vi "SimpleProducerConsumer.vi"() -> ()   [LabVIEW 2014]
doc: "This example shows a simple Producer Consumer implementation on the RasPi\ntarget. Enter Command to be sent on the String control. By pressing the\nSend button, command is sent from Producer loop and shows up on the Message Received indicator that is updated on the Consumer loop. The Count indicator updates the number of iterations the Consumer loop executes.\nSend stop command to stop both parallel loops and quit the VI."
panel:
  out "Count":i32
  out "Message Received":string
  in  "Send":bool
  in  "String":string
  # "Pass 'stop' to end program"
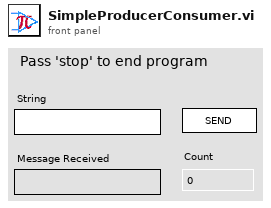
[diagram p1: front panel]
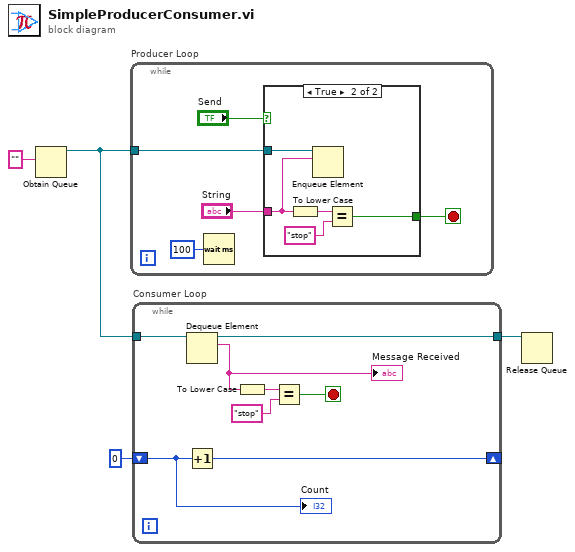
[diagram p0: block diagram]
diagram:
  n1 = Obtain Queue(element data type="") -> (queue out=w2:refnum<queue>)  [unwired: 4 in, 2 out]
  n2 = while "Producer Loop" {
    tunnel: w2 -> [w7]
    stop <- w5 stop-if-true
    n3 = Wait (ms)(milliseconds to wait=u32 100) -> ()  [unwired: 1 out]
    n4 = case shown="True" "Send" {
      tunnel: w7 -> [_ w14]
      tunnel: "String" -> [_ w13]
      tunnel: [_ w10] -> w5
      frame False {
      }
      frame True {
        n5 = To Lower Case(string=w13) -> (all lower case string=w11:string)
        n6 = Enqueue Element(queue=w14, element=w13) -> ()  [unwired: 2 in, 3 out]
        n7 = Equal?(x=w11, y="stop") -> (x = y?=w10:bool)
      }
    }
  }
  n8 = while "Consumer Loop" {
    shift-right: [w21] -> _
    shift-left: 0 -> [w15]
    tunnel: w2 -> [w22]
    tunnel: [w16] -> w1
    stop <- w17 stop-if-true
    n9 = Dequeue Element(queue=w22) -> (queue out=w16:refnum<queue>, element=w18:string)  [unwired: 2 in, 2 out]
    "Message Received" <- w18
    n10 = Increment(x=w15) -> (x+1=w21:i32)
    n11 = To Lower Case(string=w18) -> (all lower case string=w20:string)
    n12 = Equal?(x=w20, y="stop") -> (x = y?=w17:bool)
    "Count" <- w15
  }
  n13 = Release Queue(queue=w1) -> ()  [unwired: 2 in, 3 out]
